vi "Close Sample Container Connections.vi"(8 "error in (no error)":errorcluster, 11 "Storage Line in":refnum<class "Storage Line.lvclass">) -> (0 "error out":errorcluster, 3 "Storage Line out":refnum<class "Storage Line.lvclass">)   [LabVIEW 2015, in "cRIO-Carbondioxide.lvlib" / "CO2-Actor.lvlib" / "Storage Line.lvclass"]
uses:
  Storage Line.lvclass
  Storage Line.lvclass/Storage Line.ctl
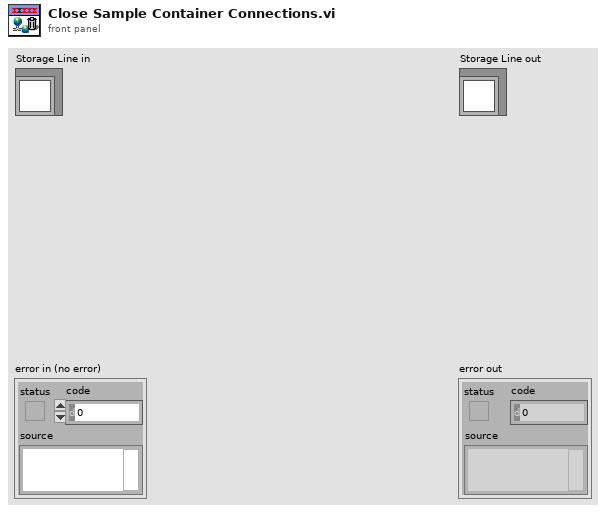
[diagram p1: front panel]
types:
  T1 = typedef "Sample Container.ctl" = cluster{"Sample In":refnum<k21>, "Sample Name":refnum<k21>, "Ti Cathode":refnum<k21>, "SampleQ":refnum<queue>}
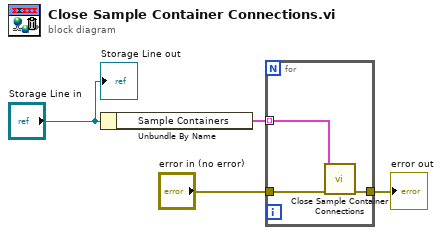
[diagram p0: block diagram]
diagram:
  n1 = Unbundle By Name("Storage Line in") -> ("Sample Containers"=w2:T1[])
  n2 = for {
    tunnel: w2 -> [w5] mode=indexing
    tunnel: "error in (no error)" -> [w7]
    tunnel: [w6] -> w1
    n3 = call "Close Sample Container Connections.vi"("error in (no error)"=w7, "Container in"=w5) -> ("error out"=w6:errorcluster)  [unwired: 8 in, 1 out]
  }
  "error out" <- w1
  "Storage Line out" <- "Storage Line in"
